vi "File Name.vi"() -> (3 "String":string)   [LabVIEW 2019]
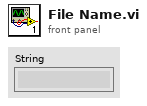
[diagram p1: front panel]
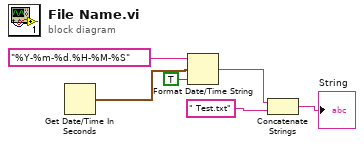
[diagram p0: block diagram]
diagram:
  n1 = Get Date/Time In Seconds() -> (seconds since 1Jan1904=w2:timestamp)
  n2 = Format Date/Time String(time format string (%c)="%Y-%m-%d.%H-%M-%S", seconds (now)=w2, UTC format=TRUE) -> (date/time string=w4:string)
  n3 = Concatenate Strings(w4, " Test.txt" ("string")) -> (→"String":string)
